vi "en_Conv.vi"(9 "en->en^2":bool, 10 "In":string) -> (2 "Out":string)   [LabVIEW 2017]
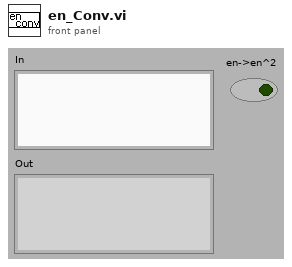
[diagram p1: front panel]
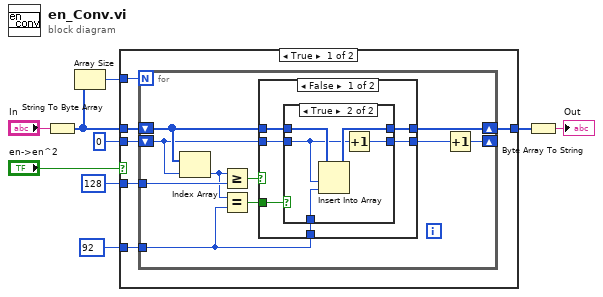
[diagram p0: block diagram]
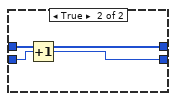
[diagram p3: hidden frame]
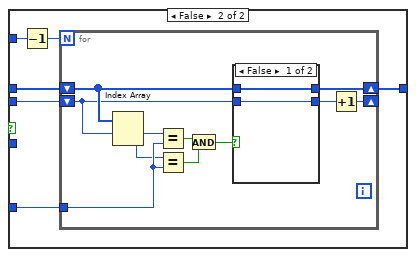
[diagram p4: hidden frame]
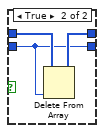
[diagram p5: hidden frame]
diagram:
  n1 = String To Byte Array(string="In") -> (unsigned byte array=w7:u8[])
  n2 = Array Size(array=w7) -> (size(s)=w8:i32)
  n3 = case shown="TRUE" "en->en^2" {
    tunnel: w8 -> [w15 w47]
    tunnel: w7 -> [w14 w46]
    tunnel: 0 -> [w13 w45]
    tunnel: u8 128 ("y") -> [w12 _]
    tunnel: u8 92 ("y") -> [w11 w44]
    tunnel: [w10 w43] -> w3
    frame True {
      n4 = for {
        N: w15 -> [_]
        shift-right: [w21] -> _
        shift-left: w13 -> [w20]
        shift-right: [w24] -> w10
        shift-left: w14 -> [w25]
        tunnel: w12 -> [w19]
        tunnel: w11 -> [w16]
        n5 = Index Array(array=w25, index=w20) -> (element=w18:u8)
        n6 = Greater Or Equal?(x=w18, y=w19) -> (x >= y?=w23:bool)
        n7 = Equal?(x=w18, y=w16) -> (x = y?=w17:bool)
        n8 = case shown="FALSE" w23 {
          tunnel: w25 -> [w31 w41]
          tunnel: [w28 w41] -> w24
          tunnel: w20 -> [w29 w40]
          tunnel: [w27 w39] -> w22
          tunnel: w17 -> [w30 _]
          tunnel: w16 -> [w26 _]
          frame False {
            n9 = case shown="TRUE" w30 {
              tunnel: w31 -> [w33 w37]
              tunnel: w29 -> [w32 w35]
              tunnel: [w33 w36] -> w28
              tunnel: [w32 w34] -> w27
              tunnel: w26 -> [_ w38]
              frame False {
              }
              frame True {
                n10 = Insert Into Array(array=w37, index=w35, new element=w38) -> (w36:u8[])
                n11 = Increment(x=w35) -> (x+1=w34:i32)
              }
            }
          }
          frame True {
            n12 = Increment(x=w40) -> (x+1=w39:i32)
          }
        }
        n13 = Increment(x=w22) -> (x+1=w21:i32)
      }
    }
    frame False {
      n14 = Decrement(x=w47) -> (x-1=w42:i32)
      n15 = for {
        N: w42 -> [_]
        shift-right: [w55] -> _
        shift-left: w45 -> [w54]
        shift-right: [w57] -> w43
        shift-left: w46 -> [w58]
        tunnel: w44 -> [w52]
        n16 = Index Array(array=w58, index #1=w54) -> (element #1=w53:u8, element #2=w48:u8)  [unwired: 1 in]
        n17 = Equal?(x=w53, y=w52) -> (x = y?=w51:bool)
        n18 = Equal?(x=w48, y=w52) -> (x = y?=w50:bool)
        n19 = And(x=w51, y=w50) -> (x .and. y?=w49:bool)
        n20 = case shown="FALSE" w49 {
          tunnel: w58 -> [w60 w63]
          tunnel: w54 -> [w59 w61]
          tunnel: [w60 w62] -> w57
          tunnel: [w59 w61] -> w56
          frame False {
          }
          frame True {
            n21 = Delete From Array(array=w63, index=w61) -> (array with subset deleted=w62:u8[])  [unwired: 1 in, 1 out]
          }
        }
        n22 = Increment(x=w56) -> (x+1=w55:i32)
      }
    }
  }
  n23 = Byte Array To String(unsigned byte array=w3) -> (string=→"Out":string)
